vi "Base INI Folder Path.vi"() -> (3 "Base Path":path)   [LabVIEW 2019]
uses:
  <vilib>/Utility/sysdir.llb/System Directory Type.ctl
panel:
  # "This is in the typedefs folder because it is a \"global constant\""
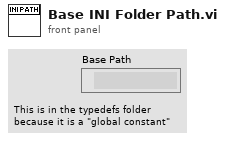
[diagram p1: front panel]
types:
  T1 = typedef "System Directory Type.ctl" = i32
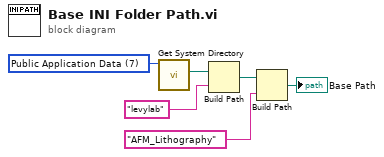
[diagram p0: block diagram]
diagram:
  w5 = T1 7 items=["User Home"=0, "User Desktop"=1, "User Documents"=2, "User Application Data"=3, "User Preferences"=4, "User Temporary"=5, "Public Documents"=6, "Public Application Data"=7, "Public Preferences"=8, "Public Cache"=13, "System Core Libraries"=9, "System Installed Libraries"=10, "Application Files"=11, "Boot Volume Root"=12] ("system directory type")
  n1 = call <vilib>:"Get System Directory.vi"("system directory type"=w5) -> ("system directory"=w6:path)  [unwired: 10 in]
  n2 = Build Path(base path=w6, name or relative path="levylab") -> (appended path=w3:path)
  n3 = Build Path(base path=w3, name or relative path="AFM_Lithography") -> (appended path=→"Base Path":path)
